vi "TriggerPointMeasurement.vi"(8 "error in":errorcluster, 9 "Set_Get":enum16{"Set", "Get"}(ring)=enum."Get", 11 "in":T1) -> (0 "error out":errorcluster, 3 "out":T1)   [LabVIEW 2010]
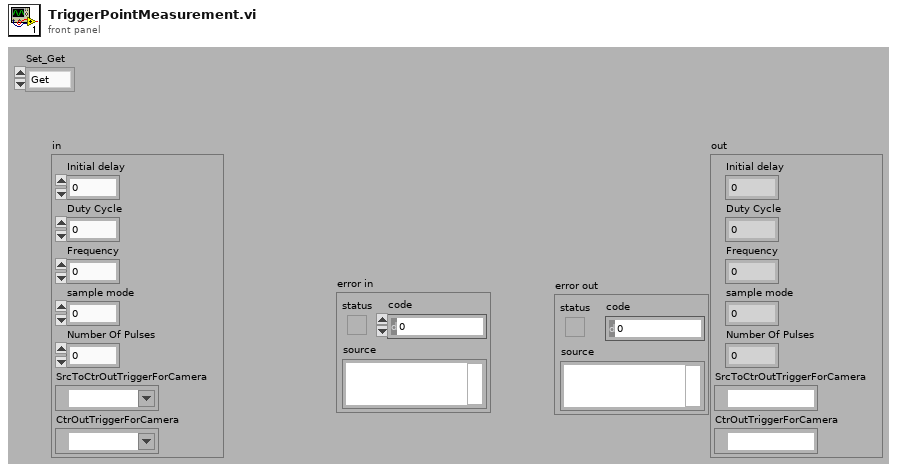
[diagram p1: front panel]
types:
  T1 = cluster{"Initial delay":dbl, "Duty Cycle":dbl, "Frequency":dbl, "sample mode":i32, "Number Of Pulses":i32, "SrcToCtrOutTriggerForCamera":tag, "CtrOutTriggerForCamera":tag}
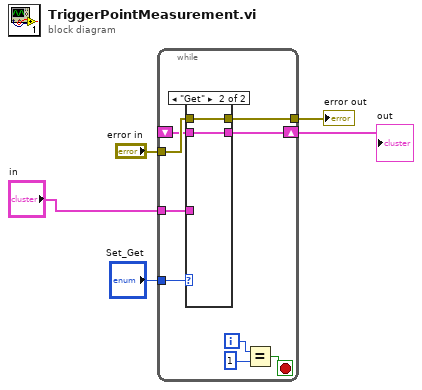
[diagram p0: block diagram]
diagram:
  n1 = while {
    tunnel: "Set_Get" -> [w14]
    tunnel: "error in" -> [w10]
    tunnel: [w9] -> w4
    tunnel: "in" -> [w8]
    shift-right: [w7] -> w1
    shift-left: _ -> [w6]
    i -> [w11]
    stop <- w12 stop-if-true
    n2 = case shown="\"Get\"" w14 {
      tunnel: w10 -> [w16 w18]
      tunnel: [w16 w18] -> w9
      tunnel: w8 -> [w15 _]
      tunnel: [w15 w17] -> w7
      tunnel: w6 -> [_ w17]
      frame "Set", Default {
      }
      frame "Get" {
      }
    }
    n3 = Equal?(x=w11, y=1) -> (x = y?=w12:bool)
  }
  "error out" <- w4
  "out" <- w1
